vi "CSP_reverseEigenvalues.vi"(8 "Eigenvectors in":T1, 9 "Eigenvalues in":cdb[](array[numeric])) -> (2 "Reversed Eigenvectors":T1, 3 "Reversed Eigenvalues":cdb[](array[numeric]))   [LabVIEW 2016, in "Spatial Pattern Filter.lvlib"]
uses:
  <vilib>/Analysis/Matrix/Datatypes/ComplexMatrix.ctl
  <vilib>/Analysis/Matrix/Numeric/Conversions/Array To Matrix - CA2.vi
  Spatial Pattern Filter.lvlib
  <vilib>/Analysis/Matrix/NI_Matrix.lvlib
panel:
  # "This VI is a part of BCI Design library, http://www.ru-bci.org \nCopyright © 2020, Sotnikov Peter, All rights reserved. License: GNU GPLv3"
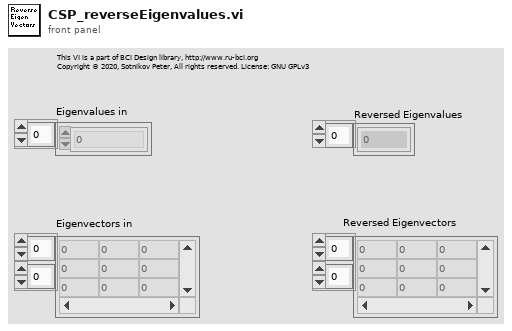
[diagram p1: front panel]
types:
  T1 = typedef "NI_Matrix.lvlib/ComplexMatrix.ctl" = cdb[][]
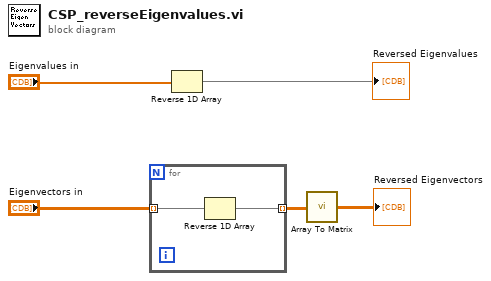
[diagram p0: block diagram]
diagram:
  n1 = for {
    tunnel: "Eigenvectors in" -> [w7] mode=indexing
    tunnel: [w6] -> w2 mode=indexing
    n2 = Reverse 1D Array(array=w7) -> (reversed array=w6:cdb[])
  }
  n3 = Reverse 1D Array(array="Eigenvalues in") -> (reversed array=→"Reversed Eigenvalues":cdb[])
  n4 = call-poly <vilib>:"Array To Matrix.vi"("Complex 2D Array"=w2) -> ("Complex Matrix"=→"Reversed Eigenvectors":T1)
